vi "Test Add Clears Redo.vi"(8 "error in":errorcluster, 11 "Test Case In":refnum<class "History Tests.lvclass">) -> (0 "error out":errorcluster, 3 "Test Case Out":refnum<class "History Tests.lvclass">)   [LabVIEW 2020, in "History Tests.lvclass"]
uses:
  History Tests.lvclass
  History Tests.lvclass/History Tests.ctl
  d374c4ae-0456-4ebf-b145-8753cc394ed2.vi
  resource/plugins/NIIconEditor/History/History/History.lvclass
  5d03536d-b951-4893-9e85-05bb1b57c72f.vi
panel:
  out "State After Redo":string
  out "State After Adding":string
  out "Undo State Outputs":string[](array[string])
  out "State After Initial Adding":string
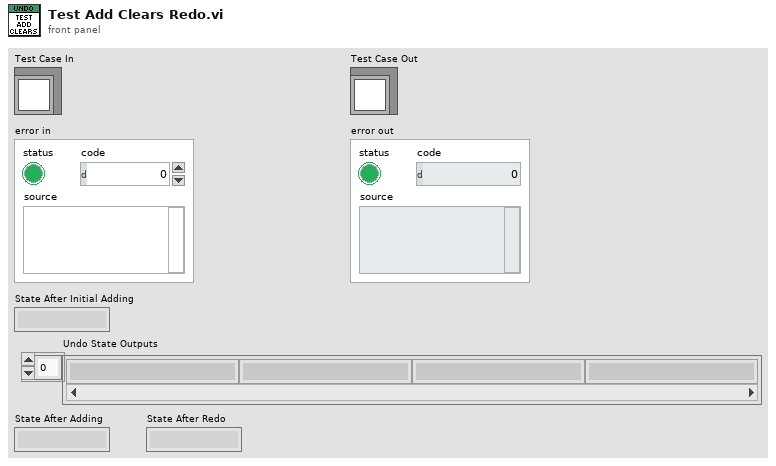
[diagram p1: front panel]
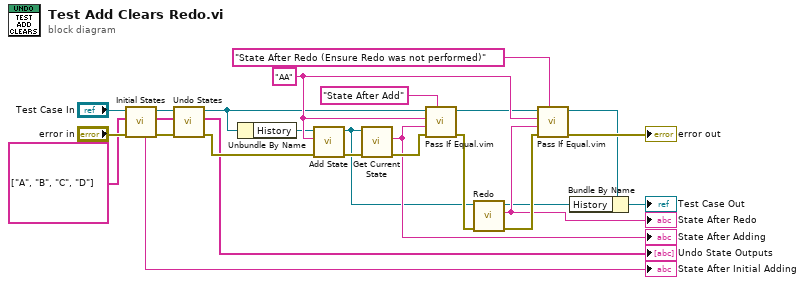
[diagram p0: block diagram]
diagram:
  w18 = "AA" ("Data in")
  n1 = call "Initial States.vi"("error in"="error in", "States"=string[] ["A", "B", "C", "D"], "Test Case In"="Test Case In") -> ("error out"=w26:errorcluster, "Expected Undo Stack"=w11:string[], "Test Case Out"=w14:refnum<class "History Tests.lvclass">, "Current State"=→"State After Initial Adding":string)  [unwired: 5 in]
  n2 = call "Undo States.vi"("error in"=w26, "Expected Undo States"=w11, "Test Case In"=w14) -> ("error out"=w25:errorcluster, "Actual Undo States"=→"Undo State Outputs":string[], "Test Case Out"=w8:refnum<class "History Tests.lvclass">)  [unwired: 6 in]
  n3 = Unbundle By Name(w8) -> ("History"=w7:refnum<class "History.lvclass">)
  n4 = call "Add State.vi"("error in"=w25, "State"=w18, "History in"=w7) -> ("error out"=w24:errorcluster, "History out"=w4:refnum<class "History.lvclass">)  [unwired: 7 in]
  n5 = call "Get Current State.vi"("error in"=w24, "History"=w4) -> ("error out"=w19:errorcluster, "Current State"=w6:string)  [unwired: 7 in, 1 out]
  "State After Adding" <- w6
  n6 = call "Pass If Equal.vim"("Description"="State After Add", "error in (no error)"=w19, "Actual"=w6, "Expected"=w18, "LUnit Test Case In"=w8) -> ("error out"=w23:errorcluster, "LUnit Test Case Out"=w9:refnum<class "History Tests.lvclass">)  [unwired: 5 in]
  n7 = call "Redo.vi"("error in"=w23, "History in"=w4) -> ("error out"=w22:errorcluster, "State"=w5:string, "History out"=w2:refnum<class "History.lvclass">)  [unwired: 7 in]
  "State After Redo" <- w5
  n8 = call "Pass If Equal.vim"("Description"="State After Redo (Ensure Redo was not performed)", "error in (no error)"=w22, "Actual"=w5, "Expected"=w18, "LUnit Test Case In"=w9) -> ("error out"=→"error out":errorcluster, "LUnit Test Case Out"=w3:refnum<class "History Tests.lvclass">)  [unwired: 5 in]
  n9 = Bundle By Name(cluster=w3, "History"=w2) -> (→"Test Case Out":refnum<class "History Tests.lvclass">)
